vi "Example Callback - Quaternion Callback.vi"(4 "Quaternion":refnum<user-event>, 5 "Event Data":T1, 6 "Control Ref":refnum<k24>, 7 "Event Common Data":T2) -> ()   [LabVIEW 2013]
uses:
  C:/tf/play/labview/Tinkerforge.dll
  Tinkerforge.dll
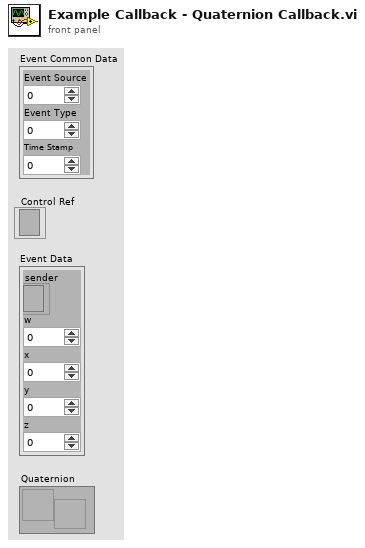
[diagram p1: front panel]
types:
  T1 = cluster{"sender":refnum<k24>, "w":i16, "x":i16, "y":i16, "z":i16}
  T2 = cluster{"Event Source":i32, "Event Type":u32, "Time Stamp":u32}
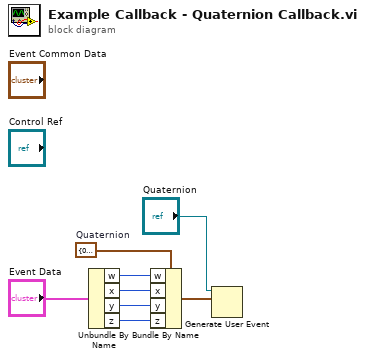
[diagram p0: block diagram]
diagram:
  w2 = cluster{"w":i16, "x":i16, "y":i16, "z":i16} {"w"=0, "x"=0, "y"=0, "z"=0}  # Quaternion
  n1 = Unbundle By Name("Event Data") -> ("w"=w7:i16, "x"=w6:i16, "y"=w5:i16, "z"=w4:i16)
  n2 = Bundle By Name(cluster=w2, "w"=w7, "x"=w6, "y"=w5, "z"=w4) -> (w1:cluster{"w":i16, "x":i16, "y":i16, "z":i16})
  n3 = Generate User Event(user event="Quaternion", event data cluster=w1) -> ()  [unwired: 2 in, 2 out]
